vi "deploy image.vi"() -> ()   [LabVIEW 2014]
panel:
  in  "Image path":path
  in  "copy":bool
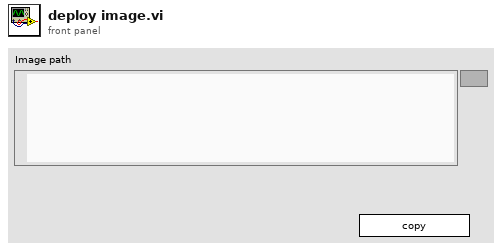
[diagram p1: front panel]
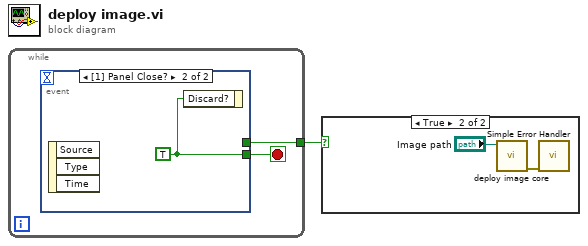
[diagram p0: block diagram]
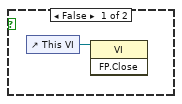
[diagram p2: hidden frame]
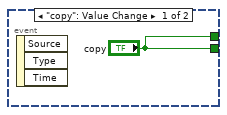
[diagram p3: hidden frame]
diagram:
  n1 = while {
    tunnel: [w2] -> w1
    stop <- w3 stop-if-true
    n2 = event shown="[1] Panel Close?" {
      selector: _ -> [_ _]
      dyn-events: _ -> [_ _]
      timeout: _ -> [_ _]
      tunnel: ["copy" w5] -> w3
      tunnel: ["copy" _] -> w2
      event "copy": Value Change {
        n3 = event-data() -> ()  [unwired: 1 in, 3 out]
      }
      event Panel Close? {
        w5 = TRUE ("Discard?")
        n4 = event-data() -> ()  [unwired: 1 in, 3 out]
        n5 = event-data("Discard?"=w5) -> ()  [unwired: 1 in, 1 out]
      }
    }
  }
  n6 = case shown="True" w1 {
    frame False {
      n7 = control-ref of="This VI"() -> (w6:refnum<vi>)
      n8 = invoke class="VI" method="FP.Close"(reference=w6) -> ()  [unwired: 2 in, 3 out]
    }
    frame True {
      n9 = call "deploy image core.vi"("image path"="Image path") -> ("error out"=w8:errorcluster)  [unwired: 10 in]
      n10 = call <vilib>:"Simple Error Handler.vi"("error in (no error)"=w8) -> ()  [unwired: 4 in, 5 out]
    }
  }
